vi "Pockels Cal-Update cal graph.vi"(7 "Function":T2(ring), 8 "error in (no error)":errorcluster, 9 "Processing Type (Interpolate)":T1, 10 "Cal table":string[][](array[string]), 11 "XYGraph in":refnum<vi>) -> (0 "error out":errorcluster, 3 "XYGraph":refnum<vi>)   [LabVIEW 2013]
uses:
  Typedefs/Pockels cal processing type.ctl
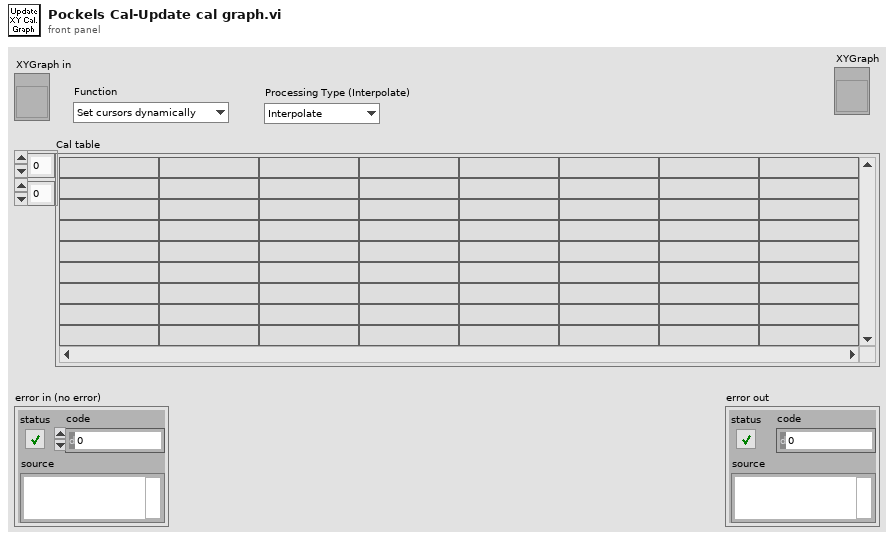
[diagram p1: front panel]
types:
  T1 = typedef "Pockels cal processing type.ctl" = enum16{"Interpolate", "Condense"}
  T2 = enum16{"Set cursors dynamically", "Set cursors from file"}
  T3 = cluster{"Start point index":i32, "End point index":i32}
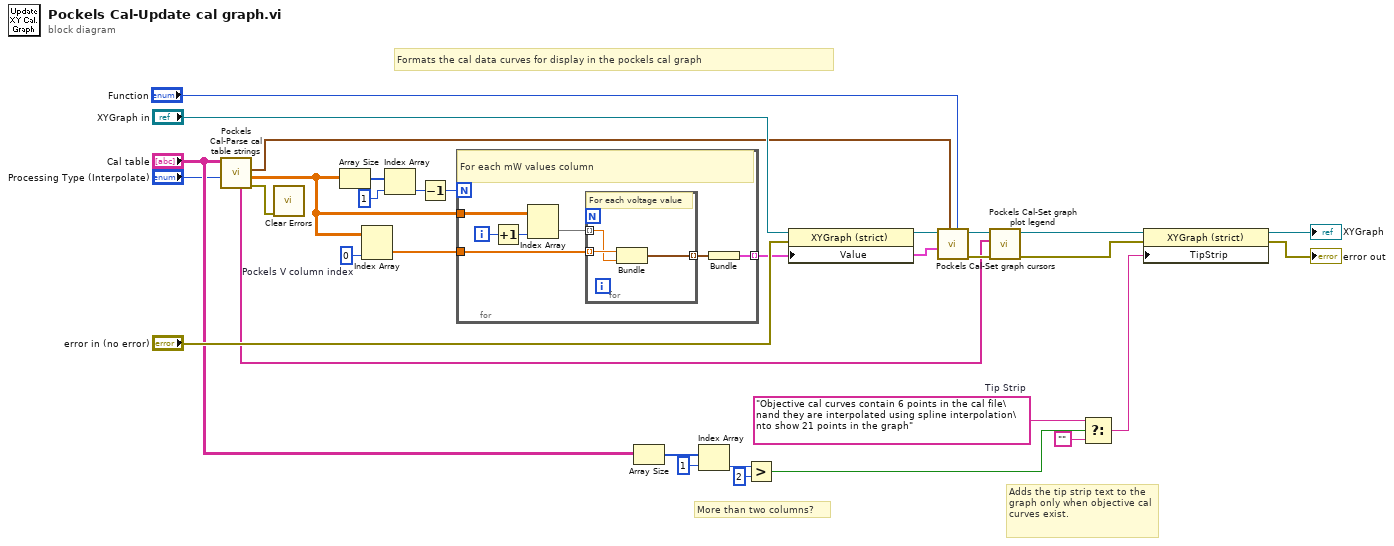
[diagram p0: block diagram]
diagram:
  w11 = "Objective cal curves contain 6 points in the cal file\nand they are interpolated using spline interpolation\nto show 21 points in the graph"  # Tip Strip
  w28 = 0  # Pockels V column index
  # "More than two columns?"
  # "Adds the tip strip text to the graph only when objective cal curves exist."
  # "Formats the cal data curves for display in the pockels cal graph"
  n1 = call "Pockels Cal-Parse cal table strings.vi"("Processing Type (Interpolate)"="Processing Type (Interpolate)", "SINGLE CAL SET (inc. headers & info)"="Cal table") -> ("error out"=w21:errorcluster, "Pockels Cal data"=w22:dbl[][], "Cal subset indexes"=w15:T3, "Cal data header"=w17:string[])  [unwired: 4 in, 2 out]
  n2 = call <vilib>:"Clear Errors.vi"("error in (no error)"=w21) -> ()  [unwired: 6 in, 1 out]
  n3 = Array Size(array=w22) -> (size(s)=w23:i32[])
  n4 = Index Array(array=w22, index (col)=w28) -> (element=w29:dbl[])  [unwired: 1 in]
  n5 = Index Array(array=w23, index=1) -> (element=w27:i32)
  n6 = Decrement(x=w27) -> (x-1=w25:i32)
  n7 = for {
    N: w25 -> [_]
    tunnel: w22 -> [w38]
    tunnel: w29 -> [w35]
    tunnel: [w33] -> w18 mode=indexing
    i -> [w37]
    # "For each mW values column"
    n8 = Increment(x=w37) -> (x+1=w32:i32)
    n9 = Index Array(array=w38, index (col)=w32) -> (element=w36:dbl[])  [unwired: 1 in]
    n10 = for {
      tunnel: w36 -> [w40] mode=indexing
      tunnel: w35 -> [w41] mode=indexing
      tunnel: [w39] -> w34 mode=indexing
      # "For each voltage value"
      n11 = Bundle("Value"=w41, "Value"=w40) -> (w39:cluster{"Value":dbl, "Value":dbl})  [unwired: 1 in]
    }
    n12 = Bundle(w34) -> (w33:cluster{cluster{"Value":dbl, "Value":dbl}[]})  [unwired: 1 in]
  }
  n13 = Array Size(array="Cal table") -> (size(s)=w13:i32[])
  n14 = Index Array(array=w13, index=1) -> (element=w9:i32)
  n15 = Greater?(x=w9, y=2) -> (0:w7:bool)
  n16 = property on="Property Node" class="XYGraph (strict)"(reference="XYGraph in", error in="error in (no error)", "Value"=w18) -> (reference out=w24:refnum<vi>)  [unwired: 1 out]
  n17 = call "Pockels Cal-Set graph cursors.vi"("Function"="Function", "Cal subset indexes"=w15, "Waveforms array"=w18, "XYGraph in"=w24) -> ("error out"=w19:errorcluster, "XYGraph out"=w20:refnum<vi>)  [unwired: 6 in]
  n18 = call "Pockels Cal-Set graph plot legend.vi"("error in (no error)"=w19, "Cal data header"=w17, "XYGraph in"=w20) -> ("error out"=w3:errorcluster, "XYGraph out"=w5:refnum<vi>)  [unwired: 6 in, 1 out]
  n19 = Select(t=w11, s=w7, f="") -> (s? t:f=w6:string)
  n20 = property class="XYGraph (strict)"(reference=w5, error in=w3, "TipStrip"=w6) -> (reference out=→"XYGraph":refnum<vi>, error out=→"error out":errorcluster)
